vi "MsgRef.vi"() -> ()   [LabVIEW 2014, in "UnitTest.lvlib" / "MsgRep.lvclass"]
uses:
  MsgRep.lvclass
  Map_lib/MapBuilder/Robot_Position.ctl
  ctl/Semantic_Voice_Array.ctl
  ctl/Semantic_Voice_Cluster.ctl
  ctl/P3AT_Panel.ctl
  ctl/Actor_Control.ctl
  ctl/Point.ctl
panel:
  in  "MapPosition_Reference":refnum<vi>
  in  "MapPosition":T1
  in  "vel_cal_Reference":refnum<vi>
  out "vel_cal":cluster{"rot_z":dbl, "lin_x":dbl}
  in  "Point_Reference":refnum<vi>
  in  "Point":T2
  in  "Actor_Control_reference":refnum<vi>
  in  "Actor_Control":T3={"JoyStick"=TRUE, "RemoteP3AT"=TRUE, "DNL_Stop"=FALSE}
  in  "P3AT_Panel_Reference":refnum<vi>
  in  "P3AT_Panel":T4={"max_vel"=0.49056603773584906, "max_rot"=0.5094339622641509, "Control_Mode"=enum."Joy"} {"max_rot" scale=0.0..1.0; "max_vel" scale=0.0..1.0}
  in  "sensor_Reference":refnum<vi>
  in  "sensor":cluster{"voltage":dbl, "motor":i8}
  in  "Semantic_Voice_Array_Reference":refnum<vi>
  out "Semantic_Voice_Cluster":T5
  in  "Semantic_Voice_Array":T6
  in  "robot_position_Reference":refnum<vi>
  in  "robot position":T7
  in  "用户事件输出":refnum<user-event>
  in  "Enum":refnum<user-event>
  in  "Text":refnum<user-event>
  in  "Stop":refnum<user-event>
  in  "通知器输出":refnum<notifier>
  in  "Test in MasterActor":string
  in  "Enum text in MasterActor":enum16{"OpenSlaveActor", "StopSlaveActor"}(ring)
  in  "Enum":T8(ring)
  in  "Network_Endpoint_Events_For_P3AT":cluster{"Connected":refnum<user-event>}
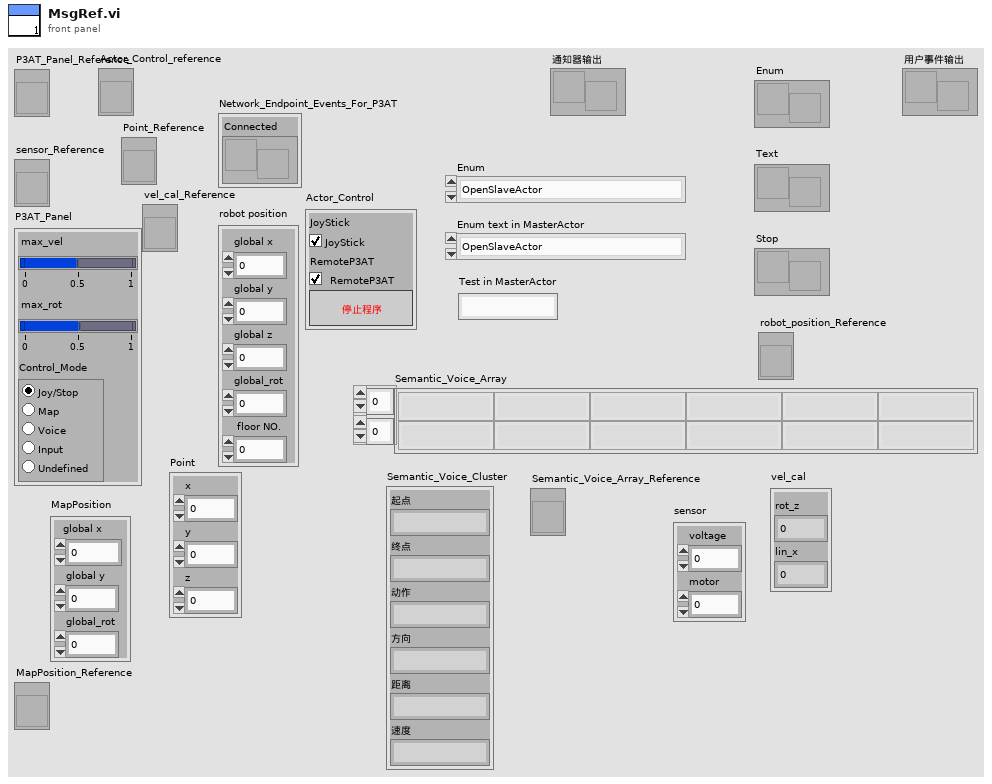
[diagram p1: front panel]
types:
  T1 = cluster{"global x":dbl, "global y":dbl, "global_rot":dbl}
  T2 = typedef "Point.ctl" = cluster{"x":dbl, "y":dbl, "z":dbl}
  T3 = typedef "Actor_Control.ctl" = cluster{"JoyStick":bool, "RemoteP3AT":bool, "DNL_Stop":bool}
  T4 = typedef "P3AT_Panel.ctl" = cluster{"max_vel":dbl, "max_rot":dbl, "Control_Mode":enum32{"Joy", "Map", "Voice", "Input", "Undefined"}}
  T5 = typedef "Semantic_Voice_Cluster.ctl" = cluster{"起点":string, "终点":string, "动作":string, "方向":string, "距离":string, "速度":string}
  T6 = typedef "Semantic_Voice_Array.ctl" = string[][]
  T7 = typedef "Robot_Position.ctl" = cluster{"global x":dbl, "global y":dbl, "global z":dbl, "global_rot":dbl, " floor NO.":dbl}
  T8 = enum16{"OpenSlaveActor", "Idle", "StopSlaveActor"}
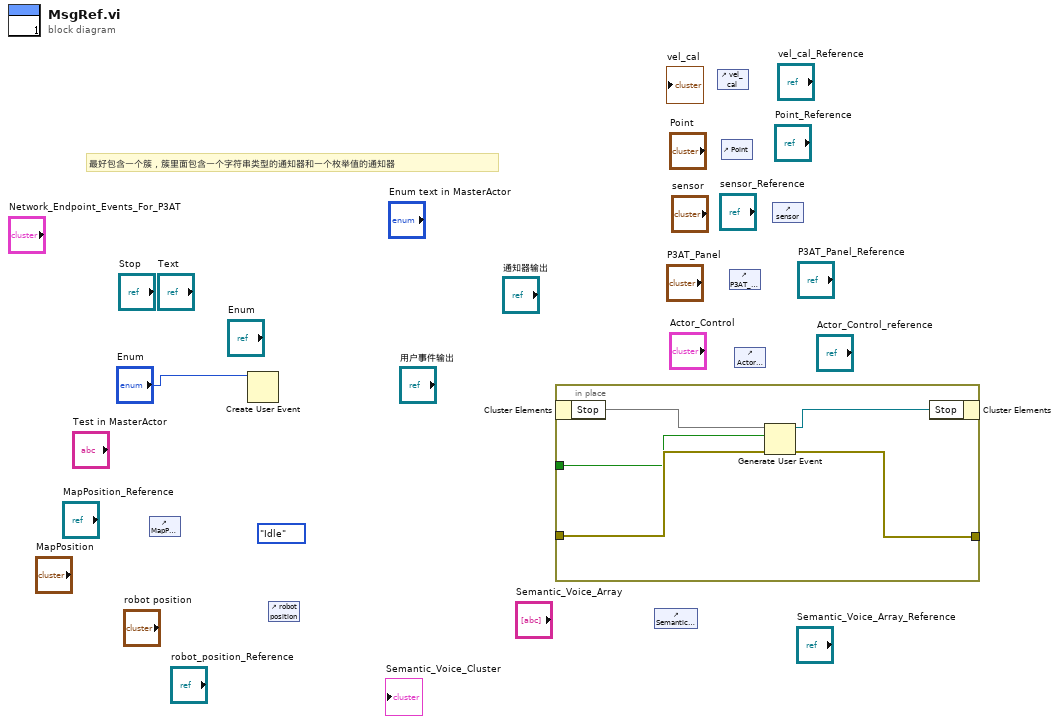
[diagram p0: block diagram]
diagram:
  (unwired) T8."Idle" ("Enum")
  # "最好包含一个簇，簇里面包含一个字符串类型的通知器和一个枚举值的通知器"
  n1 = control-ref of="MapPosition"() -> ()  [unwired: 1 out]
  n2 = Create User Event(user event datatype="Enum") -> ()  [unwired: 1 in, 2 out]
  n3 = control-ref of="robot position"() -> ()  [unwired: 1 out]
  n4 = in-place {
    in-place-border: _ -> [w4]
    in-place-border: [w3] -> _
    in-place-border: _ -> [w2]
    n5 = in-place-cluster #1() -> ("Stop"=w6)  [unwired: 1 in]
    n6 = Generate User Event(user event=w6, event data cluster=w2, error in=w4) -> (user event out=w5:refnum<user-event>, error out=w3:errorcluster)  [unwired: 1 in]
    n7 = in-place-cluster #1("Stop"=w5) -> ()  [unwired: 1 out]
  }
  n8 = control-ref of="Semantic_Voice_Array"() -> ()  [unwired: 1 out]
  n9 = control-ref of="vel_cal"() -> ()  [unwired: 1 out]
  n10 = control-ref of="Point"() -> ()  [unwired: 1 out]
  n11 = control-ref of="P3AT_Panel"() -> ()  [unwired: 1 out]
  n12 = control-ref of="Actor_Control"() -> ()  [unwired: 1 out]
  n13 = control-ref of="sensor"() -> ()  [unwired: 1 out]
